vi "SUB_WriteRTC_TIMEOUT.vi"(2 "START TIME":u32, 3 "DATA_TIME":string, 4 "telnet connection":T1) -> (0 "data out":string, 1 "OK ?":bool)   [LabVIEW 2011]
uses:
  <vilib>/addons/internet/telnet/telnet.llb/Telnet Session.ctl
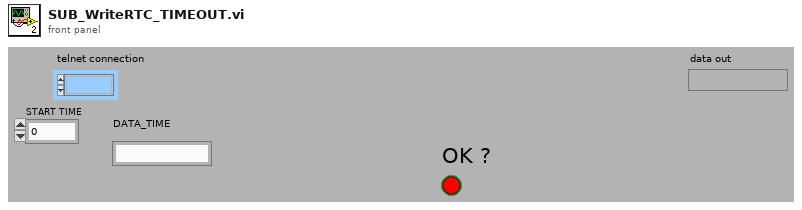
[diagram p1: front panel]
types:
  T1 = typedef "Telnet Session.ctl" = refnum<k1>
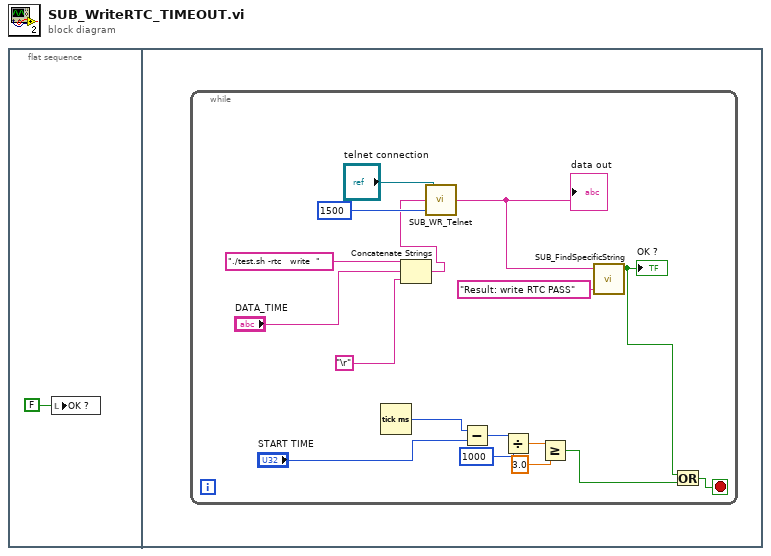
[diagram p0: block diagram]
diagram:
  n1 = flat-sequence {
    frame #0 {
      n2 = local write "OK ?"(FALSE ("OK ?")) -> ()
    }
    frame #1 {
      n3 = while {
        stop <- w10 stop-if-true
        n4 = Tick Count (ms)() -> (millisecond timer value=w8:u32)
        n5 = Concatenate Strings("./test.sh -rtc   write  ", "DATA_TIME", "\r") -> (w16:string)
        n6 = call "SUB_WR_Telnet.vi"("timeout ms"=1500, "data in"=w16, "telnet connection"="telnet connection") -> ("data out"=w14:string)  [unwired: 1 in, 1 out]
        "data out" <- w14
        n7 = Subtract(x=w8, y="START TIME") -> (x-y=w6:u32)
        n8 = Divide(x=w6, y=u32 1000) -> (x/y=w4:dbl)
        n9 = Greater Or Equal?(x=w4, y=3.0) -> (x >= y?=w2:bool)
        n10 = call "SUB_FindSpecificString.vi"("Find this String"="Result: write RTC PASS", "String data"=w14) -> ("Found"=w9:bool)  [unwired: 2 in, 1 out]
        "OK ?" <- w9
        n11 = Or(x=w9, y=w2) -> (x .or. y?=w10:bool)
      }
    }
  }
